vi "QBridge ZeroMQ.vi"() -> (0 "error":errorcluster)   [LabVIEW 2018]
uses:
  <vilib>/addons/zeromq/zmq_socket.lvclass
  <vilib>/addons/zeromq/zmq_context.lvclass
  <vilib>/addons/zeromq/socket_type.ctl
  <vilib>/addons/zeromq/socket_options.ctl
  Global_Telescopio.vi
  <vilib>/addons/zeromq/zeromq.lvlib
panel:
  out "Message to Focuser160 PULL":string
  out "Focus Status":string
  in  "QueueBaseName":string="focusQueue"
  in  "stop":bool
  # "QBRIDGE ZeroMQ"
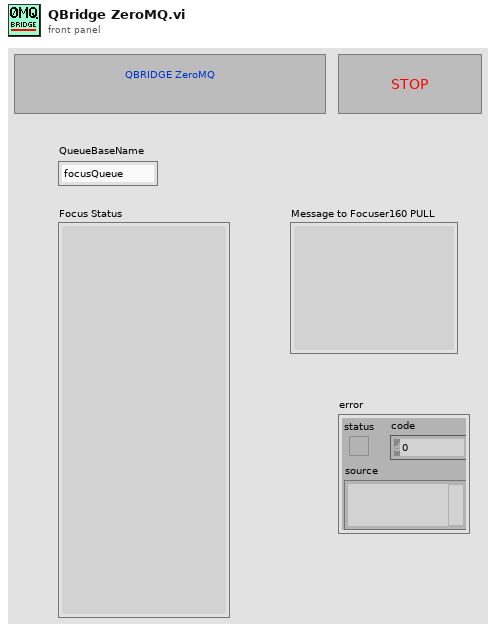
[diagram p1: front panel]
types:
  T1 = typedef "zeromq.lvlib/socket_options.ctl" = enum8{"NONE", "ZMQ_HWM", "<2>", "ZMQ_SWAP", "ZMQ_AFFINITY", "ZMQ_ROUTING_ID", "ZMQ_SUBSCRIBE", "ZMQ_UNSUBSCRIBE", "ZMQ_RATE", "ZMQ_RECOVERY_IVL", "ZMQ_MCAST_LOOP", "ZMQ_SNDBUF", "ZMQ_RCVBUF", "ZMQ_RCVMORE", "ZMQ_FD", "ZMQ_EVENTS", "ZMQ_TYPE", "ZMQ_LINGER", "ZMQ_RECONNECT_IVL", "ZMQ_BACKLOG", "ZMQ_RECOVERY_IVL_MSEC", "ZMQ_RECONNECT_IVL_MAX", "ZMQ_MAXMSGSIZE", "ZMQ_SNDHWM", "ZMQ_RCVHWM", "ZMQ_MULTICAST_HOPS", "<26>", "ZMQ_RCVTIMEO", "ZMQ_SNDTIMEO", "<29>", "<30>", "ZMQ_IPV4ONLY", "ZMQ_LAST_ENDPOINT", "ZMQ_ROUTER_MANDATORY", "ZMQ_TCP_KEEPALIVE", "ZMQ_TCP_KEEPALIVE_CNT", "ZMQ_TCP_KEEPALIVE_IDLE", "ZMQ_TCP_KEEPALIVE_INTVL", "ZMQ_TCP_ACCEPT_FILTER", "ZMQ_IMMEDIATE", "ZMQ_XPUB_VERBOSE", "ZMQ_ROUTER_RAW", "ZMQ_IPV6", "ZMQ_MECHANISM", "ZMQ_PLAIN_SERVER", "ZMQ_PLAIN_USERNAME", "ZMQ_PLAIN_PASSWORD", "ZMQ_CURVE_SERVER", "ZMQ_CURVE_PUBLICKEY", "ZMQ_CURVE_SECRETKEY", "ZMQ_CURVE_SERVERKEY", "ZMQ_PROBE_ROUTER", "ZMQ_REQ_CORRELATE", "ZMQ_REQ_RELAXED", "ZMQ_CONFLATE", "ZMQ_ZAP_DOMAIN", "ZMQ_ROUTER_HANDOVER", "ZMQ_TOS", "ZMQ_IPC_FILTER_PID", "ZMQ_IPC_FILTER_UID", "ZMQ_IPC_FILTER_GID", "ZMQ_CONNECT_ROUTING_ID", "ZMQ_GSSAPI_SERVER", "ZMQ_GSSAPI_PRINCIPAL", "ZMQ_GSSAPI_SERVICE_PRINCIPAL", "ZMQ_GSSAPI_PLAINTEXT", "ZMQ_HANDSHAKE_IVL", "<67>", "ZMQ_SOCKS_PROXY", "ZMQ_XPUB_NODROP", "ZMQ_BLOCKY", "ZMQ_XPUB_MANUAL", "ZMQ_XPUB_WELCOME_MSG", "ZMQ_STREAM_NOTIFY", "ZMQ_INVERT_MATCHING", "ZMQ_HEARTBEAT_IVL", "ZMQ_HEARTBEAT_TTL", "ZMQ_HEARTBEAT_TIMEOUT", "ZMQ_XPUB_VERBOSER", "ZMQ_CONNECT_TIMEOUT", "ZMQ_TCP_MAXRT", "ZMQ_THREAD_SAFE", "<82>", "<83>", "ZMQ_MULTICAST_MAXTPDU", "ZMQ_VMCI_BUFFER_SIZE", "ZMQ_VMCI_BUFFER_MIN_SIZE", "ZMQ_VMCI_BUFFER_MAX_SIZE", "ZMQ_VMCI_CONNECT_TIMEOUT", "ZMQ_USE_FD", "ZMQ_GSSAPI_PRINCIPAL_NAMETYPE", "ZMQ_GSSAPI_SERVICE_PRINCIPAL_NAMETYPE", "ZMQ_BINDTODEVICE", "ZMQ_ZAP_ENFORCE_DOMAIN", "ZMQ_LOOPBACK_FASTPATH", "ZMQ_METADATA", "ZMQ_MULTICAST_LOOP", "ZMQ_ROUTER_NOTIFY"}
  T2 = typedef "zeromq.lvlib/socket_type.ctl" = enum8{"ZMQ_PAIR", "ZMQ_PUB", "ZMQ_SUB", "ZMQ_REQ", "ZMQ_REP", "ZMQ_DEALER", "ZMQ_ROUTER", "ZMQ_PULL", "ZMQ_PUSH", "ZMQ_XPUB", "ZMQ_XSUB", "ZMQ_STREAM", "ZMQ_SERVER", "ZMQ_CLIENT", "ZMQ_RADIO", "ZMQ_DISH", "ZMQ_GATHER", "ZMQ_SCATTER", "ZMQ_DGRAM"}
  T3 = cluster{"broker":string, "version":string, "date":string, "hour":string, "outTemp":string, "hiTemp":string, "lowTemp":string, "outHumidity":string, "dewOut":string, "windSpeed":string, "windDirection":string, "windRun":string, "hiSpeed":string, "hiDir":string, "windChill":string, "heatIndex":string, "THWIndex":string, "THSIndex":string, "pressure":string, "rain":string, "rainRate":string, "solarRad":string, "solarEnergy":string, "hiSolarRad":string, "UVIndex":string, "UVDose":string, "hiUV":string, "headDD":string, "coolDD":string, "inTemp":string, "inHumidity":string, "inHeat":string, "inEMC":string, "inAirDensity":string, "2ndTemp":string, "2ndHumidity":string, "ET":string, "leaf":string, "windSamp":string, "windTx":string, "ISSRecept":string, "dewIn":string, "arcInt":string}
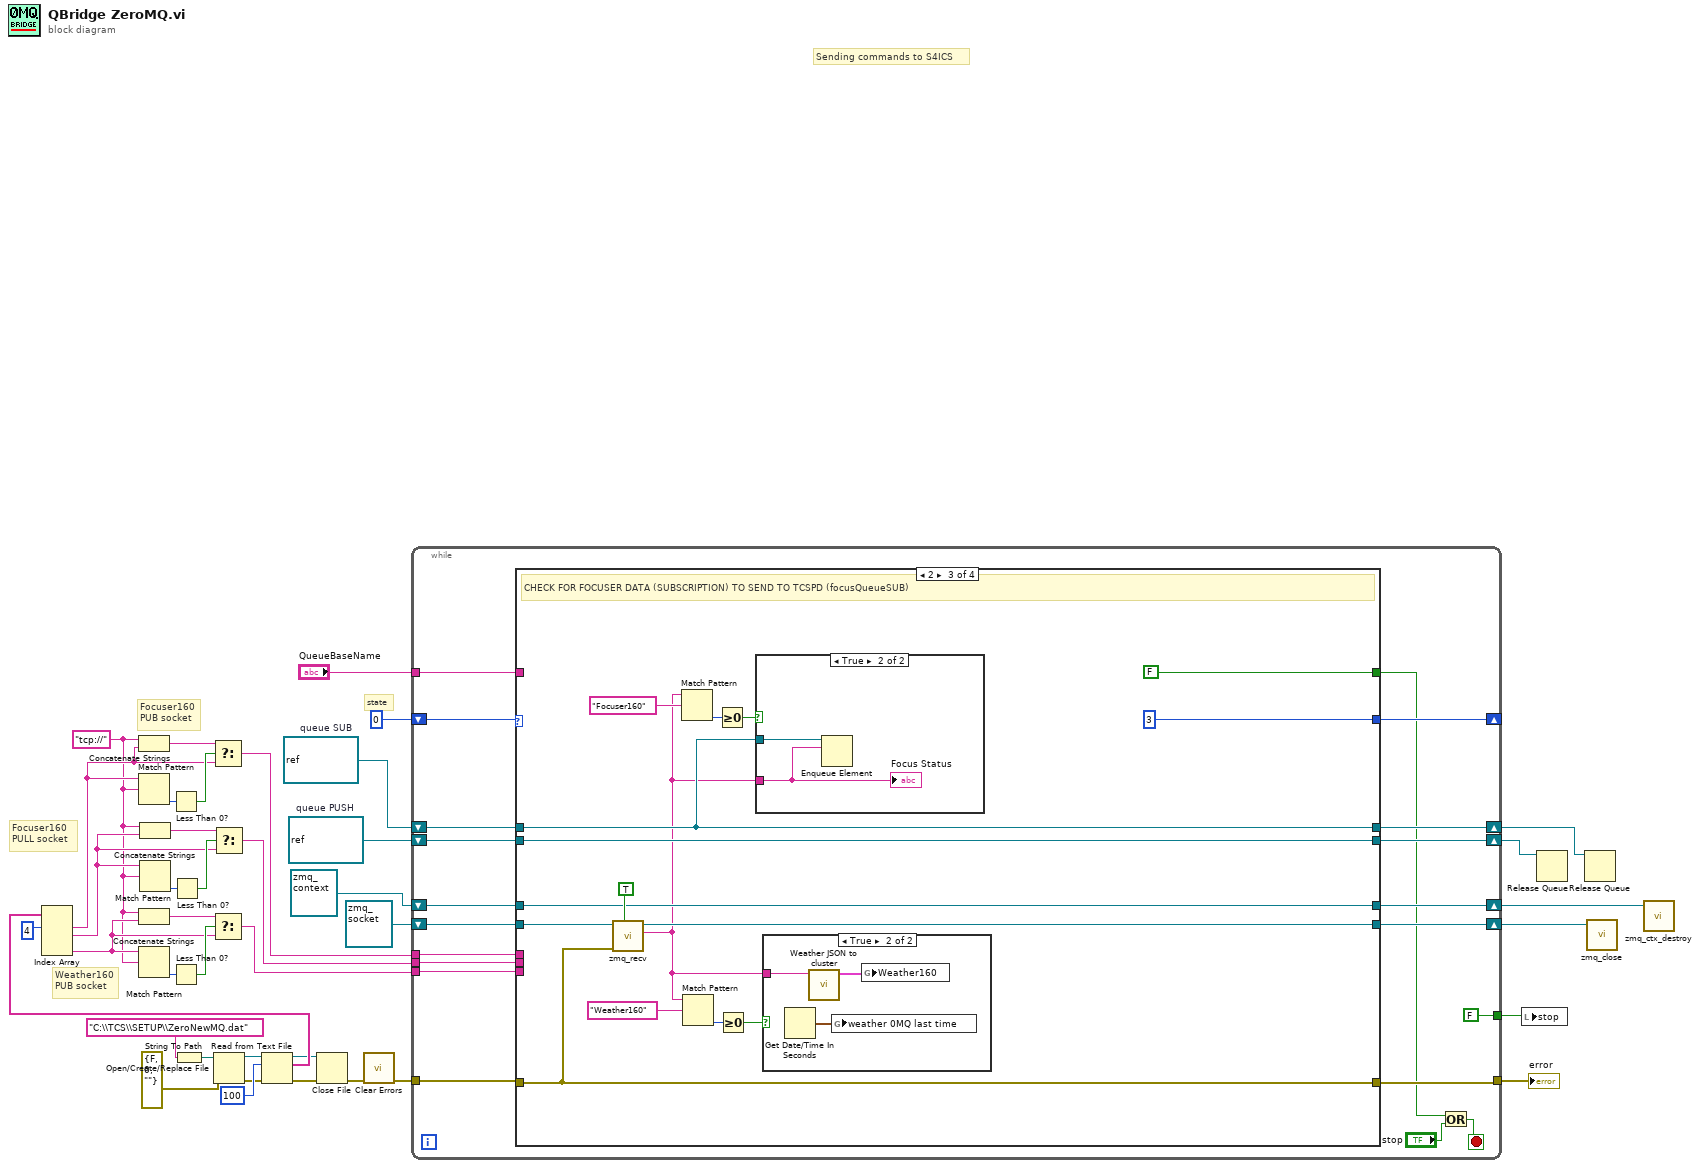
[diagram p0: block diagram]
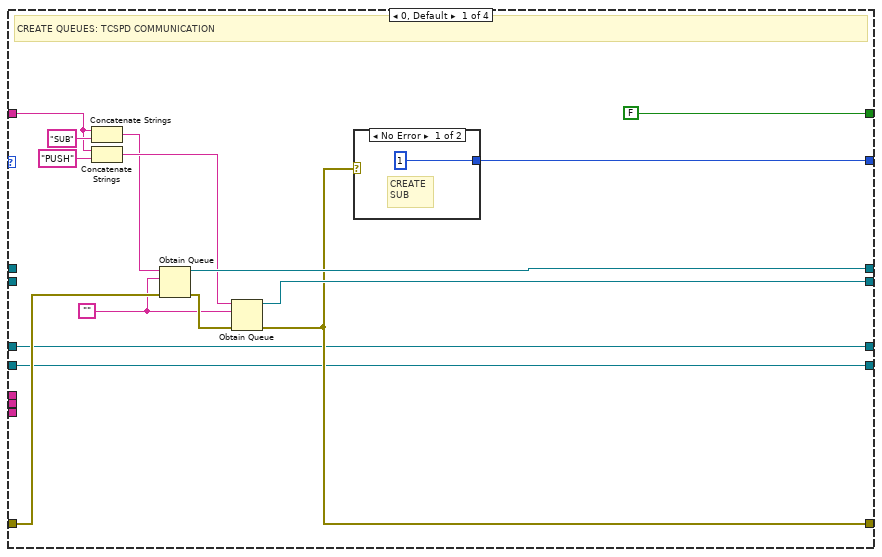
[diagram p2: hidden frame]
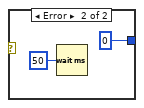
[diagram p3: hidden frame]
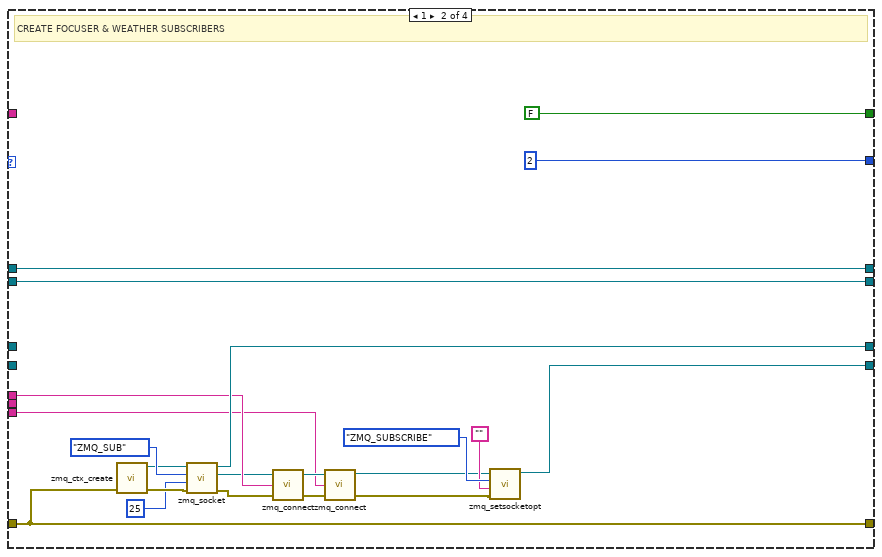
[diagram p4: hidden frame]
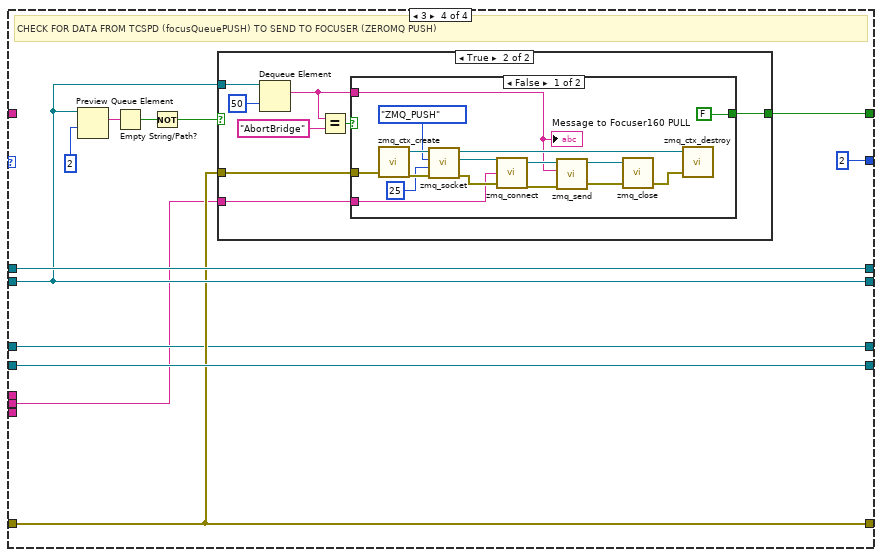
[diagram p7: hidden frame]
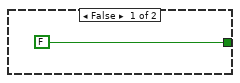
[diagram p8: hidden frame]
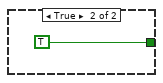
[diagram p9: hidden frame]
diagram:
  w2 = "tcp://"
  w38 = refnum<queue> refnum  # queue PUSH
  w37 = refnum<queue> refnum  # queue SUB
  # "Weather160\nPUB socket"
  # "Focuser160\nPULL socket"
  # "Focuser160\nPUB socket"
  # "state"
  # "Sending commands to S4ICS"
  n1 = String To Path(string="C:\\TCS\\SETUP\\ZeroNewMQ.dat") -> (path=w35:path)
  n2 = Open/Create/Replace File(file path (use dialog)=w35, error in=errorcluster {"status"=FALSE, "code"=0, "source"=""}) -> (refnum out=w33:refnum<file>, error out=w26:errorcluster)  [unwired: 4 in, 1 out]
  n3 = Read from Text File(file (use dialog)=w33, count=100, error in=w26) -> (refnum out=w29:refnum<file>, text=w31:string[], error out=w21:errorcluster)  [unwired: 1 in, 1 out]
  n4 = Index Array(array=w31, index #1=4 ("index")) -> (element #1=w8:string, element #2=w13:string, element #4=w3:string)  [unwired: 3 in, 1 out]
  n5 = Concatenate Strings(w2, w8) -> (w10:string)
  n6 = Match Pattern(string=w8, regular expression=w2) -> (offset past match=w9:i32)  [unwired: 1 in, 3 out]
  n7 = Concatenate Strings(w2, w3) -> (w5:string)
  n8 = Match Pattern(string=w3, regular expression=w2) -> (offset past match=w6:i32)  [unwired: 1 in, 3 out]
  n9 = Concatenate Strings(w2, w13) -> (w15:string)
  n10 = Match Pattern(string=w13, regular expression=w2) -> (offset past match=w14:i32)  [unwired: 1 in, 3 out]
  n11 = Less Than 0?(x=w9) -> (x < 0?=w11:bool)
  n12 = Less Than 0?(x=w6) -> (x < 0?=w4:bool)
  n13 = Less Than 0?(x=w14) -> (x < 0?=w16:bool)
  n14 = Select(t=w10, s=w11, f=w8) -> (s? t:f=w7:string)
  n15 = Select(t=w5, s=w4, f=w3) -> (s? t:f=w1:string)
  n16 = Select(t=w15, s=w16, f=w13) -> (s? t:f=w12:string)
  n17 = Close File(refnum=w29, error in=w21) -> (error out=w22:errorcluster)  [unwired: 1 out]
  n18 = call <vilib>:"Clear Errors.vi"("error in (no error)"=w22) -> ("error out"=w20:errorcluster)  [unwired: 5 in, 1 out]
  n19 = while {
    shift-right: [w58] -> _
    shift-left: u16 0 -> [w60]
    shift-right: [w54] -> w24
    shift-left: w37 -> [w52]
    shift-right: [w53] -> w23
    shift-left: w38 -> [w51]
    tunnel: w20 -> [w59]
    tunnel: [w57] -> w39
    tunnel: "QueueBaseName" -> [w50]
    tunnel: w7 -> [w49]
    tunnel: w12 -> [w48]
    shift-right: [w46] -> w18
    shift-left: refnum<class "zmq_socket.lvclass"> refnum ("socket out") -> [w47]
    shift-right: [w45] -> w25
    shift-left: refnum<class "zmq_context.lvclass"> refnum ("context out") -> [w43]
    tunnel: [FALSE] -> w17
    tunnel: w1 -> [w41]
    stop <- w55 stop-if-true
    n20 = case shown="2" w60 {
      tunnel: w59 -> [w72 w93 w107 w126]
      tunnel: [w73 u16 2 u16 3 u16 2] -> w58
      tunnel: [w70 w93 w107 w126] -> w57
      tunnel: [w75 w98 w112 w132] -> w54
      tunnel: [w74 w97 w115 w128] -> w53
      tunnel: w52 -> [_ w98 w112 w132]
      tunnel: w51 -> [_ w97 w115 w128]
      tunnel: w50 -> [w64 _ _ _]
      tunnel: w49 -> [_ w94 _ _]
      tunnel: w48 -> [_ _ _ w121]
      tunnel: w47 -> [w63 _ w114 w127]
      tunnel: [w63 w99 w113 w127] -> w46
      tunnel: [w61 w96 w108 w123] -> w45
      tunnel: [FALSE FALSE FALSE w124] -> w44
      tunnel: w43 -> [w61 _ w108 w123]
      tunnel: w41 -> [_ w81 _ _]
      frame 0, Default {
        w65 = ""
        # "CREATE QUEUES: TCSPD COMMUNICATION"
        n21 = Concatenate Strings(w64, "SUB" ("string")) -> (w66:string)
        n22 = Concatenate Strings(w64, "PUSH" ("string")) -> (w68:string)
        n23 = Obtain Queue(name (unnamed)=w66, element data type=w65, error in (no error)=w72) -> (queue out=w75:refnum<queue>, error out=w71:errorcluster)  [unwired: 2 in, 1 out]
        n24 = Obtain Queue(name (unnamed)=w68, element data type=w65, error in (no error)=w71) -> (queue out=w74:refnum<queue>, error out=w70:errorcluster)  [unwired: 2 in, 1 out]
        n25 = case shown="No Error" w70 {
          tunnel: [u16 1 u16 0] -> w73
          frame No Error {
            # "CREATE\nSUB"
          }
          frame Error {
            n26 = Wait (ms)(milliseconds to wait=u32 50) -> ()  [unwired: 1 out]
          }
        }
      }
      frame 1 {
        # "CREATE FOCUSER & WEATHER SUBSCRIBERS"
        n27 = call <vilib>:"zmq_ctx_create.vi"("error in"=w93) -> ("error out"=w91:errorcluster, "context out"=w90:refnum<class "zmq_context.lvclass">)  [unwired: 3 in]
        n28 = call <vilib>:"zmq_socket.vi"("error in"=w91, "linger (ms)"=25, "socket type"=socket_type."ZMQ_SUB", "context in"=w90) -> ("error out"=w88:errorcluster, "socket out"=w89:refnum<class "zmq_socket.lvclass">, "context out"=w96:refnum<class "zmq_context.lvclass">)  [unwired: 1 in]
        n29 = call <vilib>:"zmq_connect.vi"("error in"=w88, "endpoint"=w94, "socket in"=w89) -> ("error out"=w82:errorcluster, "socket out"=w83:refnum<class "zmq_socket.lvclass">)  [unwired: 1 in]
        n30 = call <vilib>:"zmq_connect.vi"("error in"=w82, "endpoint"=w81, "socket in"=w83) -> ("error out"=w80:errorcluster, "socket out"=w79:refnum<class "zmq_socket.lvclass">)  [unwired: 1 in]
        n31 = call <vilib>:"zmq_setsocketopt.vi"("error in"=w80, "value"="", "option"=socket_options."ZMQ_SUBSCRIBE", "socket in"=w79) -> ("socket out"=w99:refnum<class "zmq_socket.lvclass">)  [unwired: 2 in, 1 out]
      }
      frame 2 {
        # "CHECK FOR FOCUSER DATA (SUBSCRIPTION) TO SEND TO TCSPD (focusQueueSUB)"
        n32 = call <vilib>:"zmq_recv.vi"("no block? (F)"=TRUE, "error in"=w107, "socket in"=w114) -> ("data"=w100:string, "socket out"=w113:refnum<class "zmq_socket.lvclass">)  [unwired: 2 in, 3 out]
        n33 = Match Pattern(string=w100, regular expression="Focuser160") -> (offset past match=w106:i32)  [unwired: 1 in, 3 out]
        n34 = Match Pattern(string=w100, regular expression="Weather160") -> (offset past match=w102:i32)  [unwired: 1 in, 3 out]
        n35 = Greater Or Equal To 0?(x=w106) -> (x >= 0?=w105:bool)
        n36 = Greater Or Equal To 0?(x=w102) -> (x >= 0?=w101:bool)
        n37 = case shown="True" w105 {
          tunnel: w112 -> [_ w120]
          tunnel: w100 -> [_ w119]
          frame False {
          }
          frame True {
            n38 = Enqueue Element(queue=w120, element=w119) -> ()  [unwired: 2 in, 3 out]
            "Focus Status" <- w119
          }
        }
        n39 = case shown="True" w101 {
          tunnel: w100 -> [_ w118]
          frame False {
          }
          frame True {
            n40 = Get Date/Time In Seconds() -> (seconds since 1Jan1904=w117:timestamp)
            n41 = call "Weather JSON to cluster.vi"("JSON status"=w118) -> ("Weather160"=w116:T3)  [unwired: 10 in]
            n42 = global write "Global_Telescopio.vi" "weather 0MQ last time"(w117) -> ()
            n43 = global write "Global_Telescopio.vi" "Weather160"(w116) -> ()
          }
        }
      }
      frame 3 {
        # "CHECK FOR DATA FROM TCSPD (focusQueuePUSH) TO SEND TO FOCUSER (ZEROMQ PUSH)"
        n44 = Preview Queue Element(queue=w128, timeout in ms (-1)=2) -> (element=w131:string)  [unwired: 1 in, 3 out]
        n45 = Empty String/Path?(string/path=w131) -> (empty?=w130:bool)
        n46 = Not(x=w130) -> (.not. x?=w129:bool)
        n47 = case shown="True" w129 {
          tunnel: w128 -> [_ w141]
          tunnel: w121 -> [_ w139]
          tunnel: w126 -> [_ w140]
          tunnel: [FALSE w135] -> w124
          frame False {
          }
          frame True {
            n48 = Dequeue Element(queue=w141, timeout in ms (-1)=50) -> (element=w137:string)  [unwired: 1 in, 3 out]
            n49 = Equal?(x=w137, y="AbortBridge") -> (x = y?=w136:bool)
            n50 = case shown="False" w136 {
              tunnel: w140 -> [w152 _]
              tunnel: w139 -> [w150 _]
              tunnel: w137 -> [w145 _]
              tunnel: [FALSE TRUE] -> w135
              frame False {
                n51 = call <vilib>:"zmq_ctx_create.vi"("error in"=w152) -> ("error out"=w153:errorcluster, "context out"=w157:refnum<class "zmq_context.lvclass">)  [unwired: 3 in]
                n52 = call <vilib>:"zmq_socket.vi"("error in"=w153, "linger (ms)"=25, "socket type"=socket_type."ZMQ_PUSH", "context in"=w157) -> ("error out"=w156:errorcluster, "socket out"=w155:refnum<class "zmq_socket.lvclass">, "context out"=w147:refnum<class "zmq_context.lvclass">)  [unwired: 1 in]
                n53 = call <vilib>:"zmq_connect.vi"("error in"=w156, "endpoint"=w150, "socket in"=w155) -> ("error out"=w151:errorcluster, "socket out"=w154:refnum<class "zmq_socket.lvclass">)  [unwired: 1 in]
                n54 = call <vilib>:"zmq_send.vi"("error in"=w151, "data"=w145, "socket in"=w154) -> ("error out"=w148:errorcluster, "socket out"=w149:refnum<class "zmq_socket.lvclass">)  [unwired: 4 in]
                n55 = call <vilib>:"zmq_close.vi"("error in"=w148, "socket"=w149) -> ("error out"=w146:errorcluster)  [unwired: 3 in]
                n56 = call <vilib>:"zmq_ctx_destroy.vi"("error in"=w146, "context in"=w147) -> ()  [unwired: 3 in, 1 out]
                "Message to Focuser160 PULL" <- w145
              }
              frame True {
              }
            }
          }
        }
      }
    }
    n57 = Or(x=w44, y="stop") -> (x .or. y?=w55:bool)
  }
  "error" <- w39
  n58 = local write "stop"(w17) -> ()
  n59 = Release Queue(queue=w23) -> ()  [unwired: 2 in, 3 out]
  n60 = Release Queue(queue=w24) -> ()  [unwired: 2 in, 3 out]
  n61 = call <vilib>:"zmq_close.vi"("socket"=w18) -> ()  [unwired: 4 in, 1 out]
  n62 = call <vilib>:"zmq_ctx_destroy.vi"("context in"=w25) -> ()  [unwired: 4 in, 1 out]
